vi "Is Empty Cluster.vi"(1 "Deserialized JSON Data":refnum<class "variant.lvclass">) -> (0 "Empty Cluster?":bool)   [LabVIEW 2020, in "JKI JSON Serialization.lvlib"]
uses:
  JKI JSON Serialization.lvlib
  <userlib>/_OpenG.lib/lvdata/lvdata.llb/Array of VData to VCluster__ogtk.vi
  OpenG-Variant-Data-Library/source/library/LVData/variant.lvclass
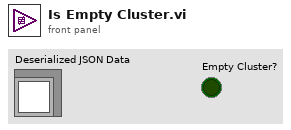
[diagram p1: front panel]
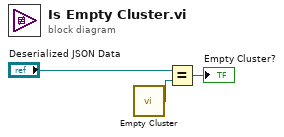
[diagram p0: block diagram]
diagram:
  n1 = call "Empty Cluster.vi"() -> ("Empty Cluster"=w2:refnum<class "variant.lvclass">)
  n2 = Equal?(x="Deserialized JSON Data", y=w2) -> (x = y?=→"Empty Cluster?":bool)
